vi "ArmLoop.vi"(11 "ArmRef":T2={"Pot"={"DevStatus"={"status"=FALSE, "code"=0, "source"=""}, "Analog Channel"=enum."Invalid", "Invert Output"=FALSE}, "ArmMotor"={"DeviceStatus"={"status"=FALSE, "code"=0, "source"=""}, "Type"=enum."PWM", "PWM"={"PWM Channel"=enum."Invalid", "DeadBand"={"Name"="", "maxPositivePwm"=0, "minPositivePwm"=0, "centerPwm"=0, "maxNegativePwm"=0, "minNegativePwm"=0, "angularRange"=0}}, "CAN"={"Device Number"=0, "Control Mode"=enum."Percent VBus", "Semaphore"=refnum, "Max Vout"=12.0, "TalonSRX Control Mode"=enum."Percent VBus"}, "Invert"=FALSE}, "Queue"=refnum, "Setpoint"=0.0, "Manual"=FALSE, "output range"={"output high"=100.0, "output low"=-0.38}, "PID gains"={"proportional gain (Kc)"=1.0, "integral time (Ti, min)"=0.01, "derivative time (Td, min)"=0.0}}) -> ()   [LabVIEW 2015, in "ArmController.lvlib"]
uses:
  ArmController.lvlib
  Typedef/ArmRef.ctl
  <vilib>/Rock Robotics/WPI/Potentiometer/WPI_PotentiometerDevRef.ctl
  <vilib>/Rock Robotics/SystemInterfaces/AI/FPGA_AIChannel.ctl
  <vilib>/Rock Robotics/WPI/MotorControl/WPI_MotorControlDeviceRef.ctl
  <vilib>/Rock Robotics/WPI/MotorControl/WPI_MotorControlType.ctl
  <vilib>/Rock Robotics/SystemInterfaces/DIO/FPGA_DIOPWMChannel.ctl
  <vilib>/Rock Robotics/WPI/PWM/WPI_PWMDeadband.ctl
  <vilib>/Rock Robotics/WPI/CAN/Jaguar/SubVIs/WPI_CANJaguar_ControlMode.ctl
  <vilib>/Rock Robotics/WPI/CAN/TalonSRX/WPI_CANTalonSRX_APIControlMode.ctl
  Typedef/MessageType.ctl
  <vilib>/Rock Robotics/Network Tables/NT Write Number.vi
  <vilib>/addons/control/pid/pid.llb/PID Advanced (DBL).vi
  <vilib>/addons/control/pid/NI_PID_pid.lvlib
panel:
  out "Chart":T1(graph)
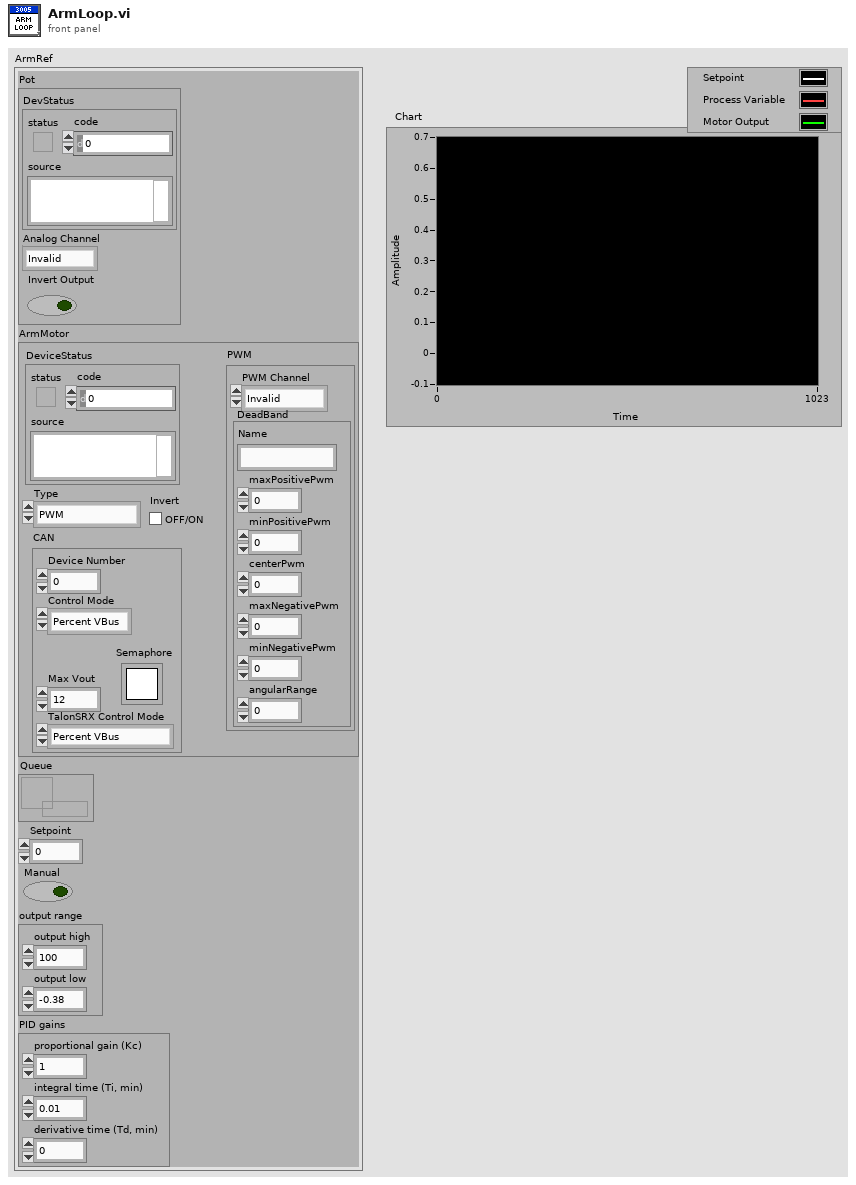
[diagram p1: front panel]
types:
  T1 = cluster{"Setpoint":dbl, "Normalized Value":dbl, "output":dbl, dbl}
  T2 = typedef "ArmController.lvlib/ArmRef.ctl" = cluster{"Pot":T3, "ArmMotor":T5, "Queue":refnum<queue>, "Setpoint":dbl, "Manual":bool, "output range":cluster{"output high":dbl, "output low":dbl}, "PID gains":cluster{"proportional gain (Kc)":dbl, "integral time (Ti, min)":dbl, "derivative time (Td, min)":dbl}}
  T3 = typedef "WPI_PotentiometerDevRef.ctl" = cluster{"DevStatus":errorcluster, "Analog Channel":T4, "Invert Output":bool}
  T4 = typedef "FPGA_AIChannel.ctl" = enum8{"AI 0", "AI 1", "AI 2", "AI 3", "AI MXP 0", "AI MXP 1", "AI MXP 2", "AI MXP 3", "Invalid"}
  T5 = typedef "WPI_MotorControlDeviceRef.ctl" = cluster{"DeviceStatus":errorcluster, "Type":T6, "PWM":cluster{"PWM Channel":T7, "DeadBand":T8}, "CAN":cluster{"Device Number":u8, "Control Mode":T9, "Semaphore":T10, "Max Vout":dbl, "TalonSRX Control Mode":T11}, "Invert":bool}
  T6 = typedef "WPI_MotorControlType.ctl" = enum16{"PWM", "CAN", "CANTalonSRX"}
  T7 = typedef "FPGA_DIOPWMChannel.ctl" = enum8{"PWM 0", "PWM 1", "PWM 2", "PWM 3", "PWM 4", "PWM 5", "PWM 6", "PWM 7", "PWM 8", "PWM 9", "PWM MXP 0", "PWM MXP 1", "PWM MXP 2", "PWM MXP 3", "PWM MXP 4", "PWM MXP 5", "PWM MXP 6", "PWM MXP 7", "PWM MXP 8", "PWM MXP 9", "Invalid"}
  T8 = typedef "WPI_PWMDeadband.ctl" = cluster{"Name":string, "maxPositivePwm":i32, "minPositivePwm":i32, "centerPwm":i32, "maxNegativePwm":i32, "minNegativePwm":i32, "angularRange":u16}
  T9 = typedef "WPI_CANJaguar_ControlMode.ctl" = enum8{"Percent VBus", "Current", "Speed", "Position", "Voltage"}
  T10 = typedef "Semaphore RefNum" = refnum<k1>
  T11 = typedef "WPI_CANTalonSRX_APIControlMode.ctl" = enum8{"Percent VBus", "Speed", "Position", "Slave", "Unchanged / Invalid", "Voltage Compensation", "Current", "Motion Profile"}
  T12 = cluster{"proportional gain (Kc)":dbl, "integral time (Ti, min)":dbl, "derivative time (Td, min)":dbl}
  T13 = typedef "ArmController.lvlib/MessageType.ctl" = cluster{"Value":dbl, "Manual Control":bool, "Auto Switch":bool}
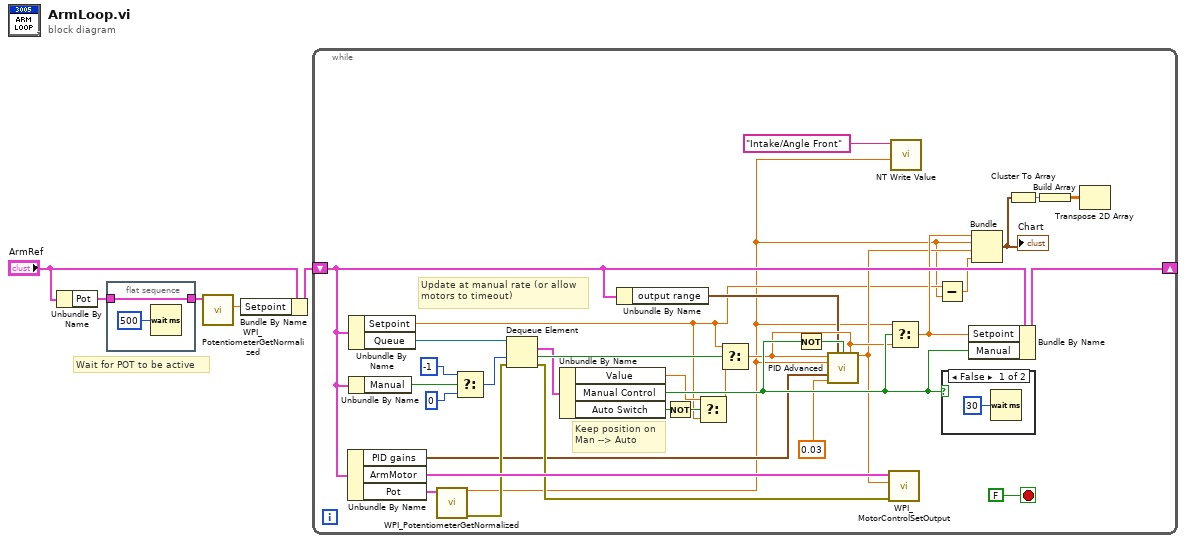
[diagram p0: block diagram]
diagram:
  # "Wait for POT to be active"
  n1 = Unbundle By Name("ArmRef") -> ("Pot"=w2:T3)
  n2 = flat-sequence {
    tunnel: w2 -> [w7]
    tunnel: [w7] -> w1
    frame #0 {
      n3 = Wait (ms)(milliseconds to wait=u32 500) -> ()  [unwired: 1 out]
    }
  }
  n4 = call <vilib>:"WPI_PotentiometerGetNormalized.vi"("PotDevRef"=w1) -> ("Normalized Value"=w3:dbl)  [unwired: 8 in, 2 out]
  n5 = Bundle By Name(cluster="ArmRef", "Setpoint"=w3) -> (w5:T2)
  n6 = while {
    shift-right: [w36] -> _
    shift-left: w5 -> [w24]
    stop <- FALSE stop-if-true
    # "Keep position on\nMan --> Auto"
    # "Update at manual rate (or allow\nmotors to timeout)"
    n7 = Unbundle By Name(w24) -> ("PID gains"=w13:T12, "ArmMotor"=w35:T5, "Pot"=w37:T3)
    n8 = Unbundle By Name(w24) -> ("Setpoint"=w14:dbl, "Queue"=w40:refnum<queue>)
    n9 = Unbundle By Name(w24) -> ("Manual"=w31:bool)
    n10 = call <vilib>:"WPI_PotentiometerGetNormalized.vi"("PotDevRef"=w37) -> ("error out"=w30:errorcluster, "Normalized Value"=w11:dbl)  [unwired: 8 in, 1 out]
    n11 = Select(t=-1 ("timeout in ms (-1)"), s=w31, f=0 ("timeout in ms (-1)")) -> (s? t:f=w32:i32)
    n12 = Dequeue Element(queue=w40, timeout in ms (-1)=w32, error in (no error)=w30) -> (element=w38:T13, timed out?=w39:bool, error out=w29:errorcluster)  [unwired: 1 out]
    n13 = Unbundle By Name(w38) -> ("Value"=w17:dbl, "Manual Control"=w28:bool, "Auto Switch"=w19:bool)
    n14 = Unbundle By Name(w24) -> ("output range"=w20:cluster{"output high":dbl, "output low":dbl})
    n15 = Not(x=w19) -> (.not. x?=w16:bool)
    n16 = Select(t=w17, s=w16, f=w14) -> (s? t:f=w18:dbl)
    n17 = Select(t=w14, s=w39, f=w18) -> (s? t:f=w27:dbl)
    n18 = Not(x=w28) -> (.not. x?=w21:bool)
    n19 = call-poly <vilib>:"PID Advanced.vi"("setpoint"=w27, "output range"=w20, "auto? (T)"=w21, "manual control"=w27, "process variable"=w11, "PID gains"=w13, "dt (s)"=0.03) -> ("output"=w22:dbl)  [unwired: 7 in, 1 out]
    n20 = call <vilib>:"WPI_MotorControlSetOutput.vi"("error in (no error)"=w29, "Output"=w22, "MotorControlDevRef"=w35) -> ()  [unwired: 6 in, 3 out]
    n21 = Select(t=w11, s=w28, f=w27) -> (s? t:f=w23:dbl)
    n22 = call-poly <vilib>:"NT Write Value.vi"("Numeric"=w11, "Name"="Intake/Angle Front") -> ()  [unwired: 9 in, 1 out]
    n23 = Subtract(x=w14, y=w11) -> (x-y=w15:dbl)
    n24 = case shown="False" w28 {
      frame False {
        n25 = Wait (ms)(milliseconds to wait=u32 30) -> ()  [unwired: 1 out]
      }
      frame True {
      }
    }
    n26 = Bundle By Name(cluster=w24, "Setpoint"=w23, "Manual"=w28) -> (w36:T2)
    n27 = Bundle("Setpoint"=w23, "Normalized Value"=w11, "output"=w22, w15) -> (w10:T1)  [unwired: 1 in]
    "Chart" <- w10
    n28 = Cluster To Array(cluster=w10) -> (array=w9:dbl[])
    n29 = Build Array(w9) -> (w8:dbl[][])
    n30 = Transpose 2D Array(2D array=w8) -> ()  [unwired: 1 out]
  }
